vi "ADIS16470 Read Multiple Registers.vi"(8 "error in (no error)":errorcluster, 10 "Registers":T3[](array[typedef]) items=["Reserved", "_Reserved", "DIAG_STAT", "_DIAG_STAT", "X_GYRO_LOW", "_X_GYRO_LOW", "X_GYRO_OUT", "_X_GYRO_OUT", "Y_GYRO_LOW", "_Y_GYRO_LOW", ""], 11 "SPIDevRef":T1) -> (0 "error out":errorcluster, 3 "Values":u16[](array[numeric]))   [LabVIEW 2018]
uses:
  Typedef/ADIS16470 Register.ctl
  <vilib>/Rock Robotics/WPI/SPI/WPI_SPIDevRef.ctl
  <vilib>/Rock Robotics/SystemInterfaces/spilib/spi_bus.ctl
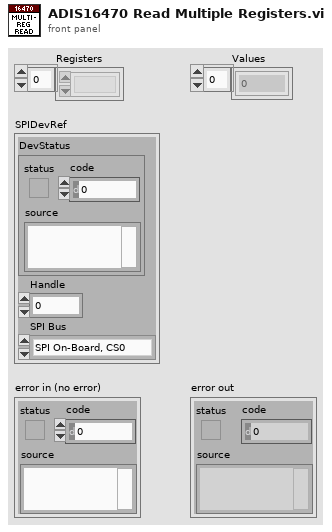
[diagram p1: front panel]
types:
  T1 = typedef "WPI_SPIDevRef.ctl" = cluster{"DevStatus":errorcluster, "Handle":i32, "SPI Bus":T2}
  T2 = typedef "spi_bus.ctl" = enum16{"SPI On-Board, CS0", "SPI On-Board, CS1", "SPI On-Board, CS2", "SPI On-Board, CS3", "SPI MXP", "Invalid"}
  T3 = typedef "ADIS16470 Register.ctl" = u8
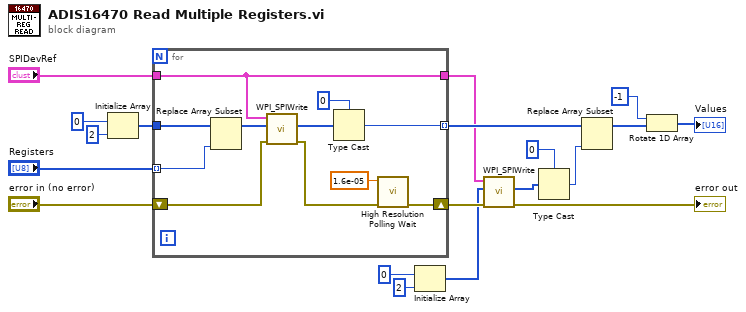
[diagram p0: block diagram]
diagram:
  n1 = Initialize Array(u8 0 ("element"), 2 ("dimension size")) -> (w12:u8[])
  n2 = for {
    tunnel: w12 -> [w26]
    tunnel: "Registers" -> [w27] mode=indexing
    tunnel: "SPIDevRef" -> [w23]
    shift-right: [w21] -> w6
    shift-left: "error in (no error)" -> [w25]
    tunnel: [w24] -> w9 mode=indexing
    tunnel: [w23] -> w7
    n3 = Replace Array Subset(array=w26, new element=w27) -> (w28:u8[])  [unwired: 1 in]
    n4 = call <vilib>:"WPI_SPIWrite.vi"("error in (no error)"=w25, "Data To Send"=w28, "SPIDevRef"=w23) -> ("error out"=w22:errorcluster, "Received Data"=w29:u8[])  [unwired: 7 out]
    n5 = Type Cast(type=u16 0, x=w29) -> (*(type *) &x=w24:u16)
    n6 = call <vilib>:"High Resolution Polling Wait.vi"("error in (no error)"=w22, "seconds to wait"=1.6e-05) -> ("error out"=w21:errorcluster)  [unwired: 9 in]
  }
  n7 = Initialize Array(u8 0 ("element"), 2 ("dimension size")) -> (w2:u8[])
  n8 = call <vilib>:"WPI_SPIWrite.vi"("error in (no error)"=w6, "Data To Send"=w2, "SPIDevRef"=w7) -> ("error out"=→"error out":errorcluster, "Received Data"=w1:u8[])  [unwired: 7 out]
  n9 = Type Cast(type=u16 0, x=w1) -> (*(type *) &x=w16:u16)
  n10 = Replace Array Subset(array=w9, new element=w16) -> (w15:u16[])  [unwired: 1 in]
  n11 = Rotate 1D Array(1:w15, 2:-1 ("n")) -> (0:→"Values":u16[])
